vi "Check Status (No Objects).vi"(8 "error in (no error)":errorcluster, 11 "Cluster In":T13={"Channel Names"=[], "Channel Units"=[], "Most Recent Data Points"=[], "History Buffers"=[], "Ring Buffers"=[], "Averaging"=enum."On", "Units"=enum."Watt", "Measuring rate"=enum."Hold", "Unit Range"=enum."10 mW (+10 dBm)", "Calibration Factor"=-26.67, "Auto Ranging?"=enum."Off"}) -> (0 "error out":errorcluster, 1 "Status":string, 2 "Ready?":bool, 3 "Cluster Out":T13={"Channel Names"=[], "Channel Units"=[], "Most Recent Data Points"=[], "History Buffers"=[], "Ring Buffers"=[], "Averaging"=enum."On", "Units"=enum."Watt", "Measuring rate"=enum."Hold", "Unit Range"=enum."10 mW (+10 dBm)", "Calibration Factor"=-26.67, "Auto Ranging?"=enum."Off"})   [LabVIEW 2009]
doc: "(Dynamic) Check if the instrument is powered on and update its member fields with the instrument's current status. Optionally return a text status message."
uses:
  Utility Classes/Readable/Channel Names.ctl
  Utility Classes/Readable/Channel Units.ctl
  Utility Classes/Readable/Data Points.ctl
  Utility Classes/Readable/Data Point.ctl
  Utility Classes/Readable/Time.ctl
  Utility Classes/Readable/X.ctl
  Utility Classes/Readable/TX Graph.ctl
  Anritsu Power Meter/Public/Averaging control.ctl
  Anritsu Power Meter/Public/Display control.ctl
  Anritsu Power Meter/Public/Measuring rate control.ctl
  Anritsu Power Meter/Public/Range control watts and dBm.ctl
  Anritsu Power Meter/Public/Auto Range control.ctl
  Global/GPIB Numbers.vi
  <vilib>/regexp/Match Regular Expression.xnode
  Utility Classes/Readable/Readable.lvclass
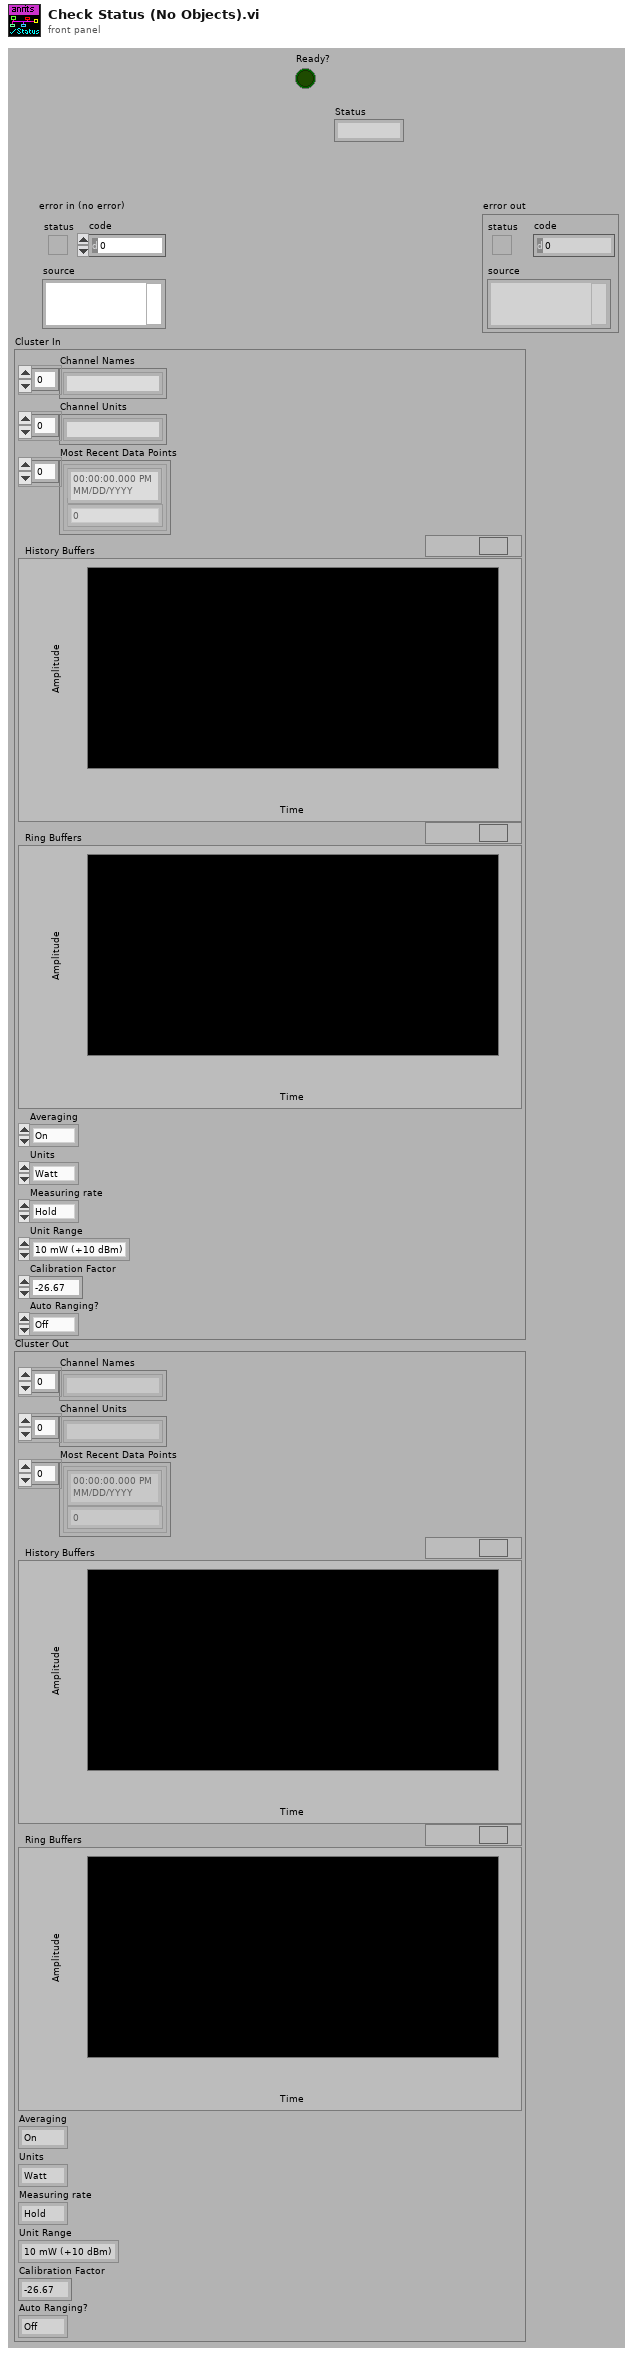
[diagram p1: front panel]
types:
  T1 = typedef "Readable.lvclass/Channel Names.ctl" = string[]
  T2 = typedef "Readable.lvclass/Channel Units.ctl" = string[]
  T3 = typedef "Readable.lvclass/Data Points.ctl" = T4[]
  T4 = typedef "Readable.lvclass/Data Point.ctl" = cluster{"t":T5, "x":T6}
  T5 = typedef "Readable.lvclass/Time.ctl" = timestamp
  T6 = typedef "Readable.lvclass/X.ctl" = dbl
  T7 = typedef "Readable.lvclass/TX Graph.ctl" = cluster{"Data Points":cluster{"t":timestamp, "x":dbl}[]}[]
  T8 = typedef "Averaging control.ctl" = enum16{"On", "Off"}
  T9 = typedef "Display control.ctl" = enum16{"Watt", "dBm", "dB (REL)"}
  T10 = typedef "Measuring rate control.ctl" = enum16{"Hold", "Free Run", "Exit Trigger"}
  T11 = typedef "Range control watts and dBm.ctl" = enum16{"10 mW (+10 dBm)", "1 mW (0 dBm)", "100 uW (-10 dBm)", "10 uW (-20 dBm)", "1 uW (-30 dBm)", "100 nW (-40 dBm)", "10 nW (-50 dBm)", "1 nW (-60 dBm)", "100 pW (-70 dBm)", "10 pW (-80 dBm)"}
  T12 = typedef "Auto Range control.ctl" = enum16{"Off", "On"}
  T13 = cluster{"Channel Names":T1, "Channel Units":T2, "Most Recent Data Points":T3, "History Buffers":T7, "Ring Buffers":T7, "Averaging":T8, "Units":T9, "Measuring rate":T10, "Unit Range":T11, "Calibration Factor":dbl, "Auto Ranging?":T12}
  T14 = cluster{"Name":string, "bus":dbl, "GPIB":dbl, "GPIB as string":string, "byte":i32, "VISA Resource Name":refnum<visa-resource-name>}
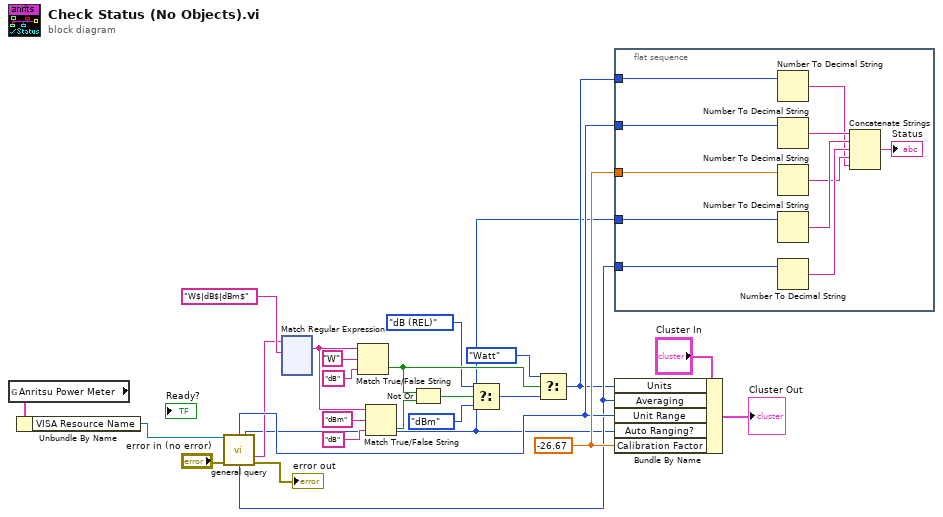
[diagram p0: block diagram]
diagram:
  w25 = -26.67 ("Calibration Factor")
  n1 = global read "GPIB Numbers.vi" "Anritsu Power Meter"() -> (w2:T14)
  n2 = Unbundle By Name(w2) -> ("VISA Resource Name"=w1:refnum<visa-resource-name>)
  n3 = call "general query.vi"("VISA resource name"=w1, "error in (no error)"="error in (no error)") -> ("Range W and dBm"=w24:T11, "Units"=w9:string, "Averaging"=w23:T8, "Auto Ranging?"=w7:T12, "error out"=→"error out":errorcluster)  [unwired: 5 in, 4 out]
  n4 = xnode "Match Regular Expression"("input string"=w9, "regular expression"="W$|dB$|dBm$") -> ("whole match"=w19:string)  [unwired: 4 in, 4 out]
  n5 = Match True/False String(2:"dB" ("false string"), 3:"W", 4:w19) -> (0:w15:bool)  [unwired: 1 out]
  n6 = Match True/False String(2:"dB" ("false string"), 3:"dBm" ("true string"), 4:w19) -> (0:w16:bool)  [unwired: 1 out]
  n7 = Not Or(1:w16, 2:w15) -> (0:w13:bool)
  n8 = Select(t=Display_control."dB (REL)" ("Display Units"), s=w13, f=Display_control."dBm" ("Display Units")) -> (s? t:f=w10:T9)
  n9 = Select(t=Display_control."Watt" ("Display Units"), s=w15, f=w10) -> (s? t:f=w8:T9)
  n10 = flat-sequence {
    tunnel: w23 -> [w34]
    tunnel: w25 -> [w36]
    tunnel: w8 -> [w33]
    tunnel: w24 -> [w35]
    tunnel: w7 -> [w26]
    frame #0 {
      n11 = Number To Decimal String(number=w33) -> (decimal integer string=w28:string)  [unwired: 1 in]
      n12 = Number To Decimal String(number=w35) -> (decimal integer string=w32:string)  [unwired: 1 in]
      n13 = Number To Decimal String(number=w36) -> (decimal integer string=w29:string)  [unwired: 1 in]
      n14 = Number To Decimal String(number=w26) -> (decimal integer string=w31:string)  [unwired: 1 in]
      n15 = Number To Decimal String(number=w34) -> (decimal integer string=w30:string)  [unwired: 1 in]
      n16 = Concatenate Strings(w32, w31, w30, w29, w28) -> (→"Status":string)
    }
  }
  n17 = Bundle By Name(cluster="Cluster In", "Units"=w8, "Averaging"=w23, "Unit Range"=w24, "Auto Ranging?"=w7, "Calibration Factor"=w25) -> (→"Cluster Out":T13)
